vi "Read_Stream_Data_EMG_Control.vi"(8 "error in (no error)":errorcluster, 11 "endpoint in":refnum<k21>) -> (0 "error out":errorcluster, 1 "EMG control":T1(ring), 2 "Reset to zero position?":bool, 3 "endpoint out":refnum<k21>, 4 "Motor speed (bit)":u8, 5 "Enabled motor?":bool)   [LabVIEW 2015]
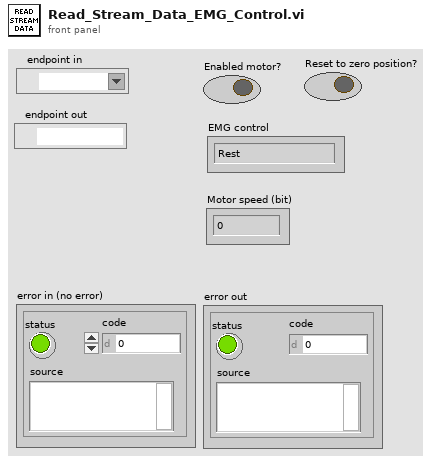
[diagram p1: front panel]
types:
  T1 = enum16{"Rest", "Biceps contracted", "Triceps contracted"}
  T2 = cluster{"Enable?":bool, "Reset?":bool, "EMG control":enum16{"Rest", "Biceps contracted", "Triceps contracted"}, "Motor speed":u8}
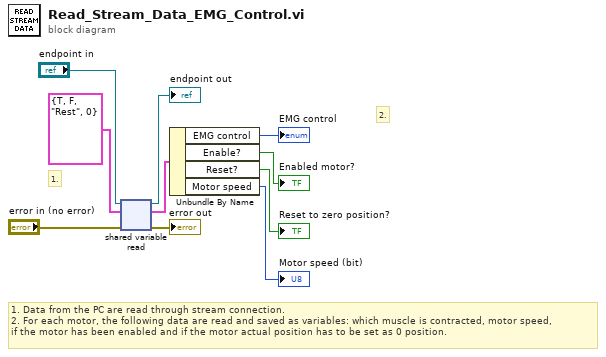
[diagram p0: block diagram]
diagram:
  # "2."
  # "1."
  # "1. Data from the PC are read through stream connection.\n2. For each motor, the following data are read and saved as variables: which muscle is contracted, motor speed,\nif the motor has been enabled and if the motor actual position has to be set as 0 position."
  n1 = shared-variable-read("endpoint in", "error in (no error)", T2 {"Enable?"=TRUE, "Reset?"=FALSE, "EMG control"=enum."Rest", "Motor speed"=0} ("data in")) -> (→"endpoint out":refnum<k21>, →"error out":errorcluster, w10:T2)  [unwired: 1 in, 1 out]
  n2 = Unbundle By Name(w10) -> ("EMG control"=→"EMG control":T1, "Enable?"=→"Enabled motor?":bool, "Reset?"=→"Reset to zero position?":bool, "Motor speed"=→"Motor speed (bit)":u8)
